vi "log_notifier.vi"(11 "NotifierReferences":T1) -> ()   [LabVIEW 2013]
doc: "Reads a log file and sends read data to the notifier once per second"
uses:
  Data/TypeDefs/Notifiers.ctl
  Data/TypeDefs/UTM Location.ctl
  Data/TypeDefs/Sail Set Suggestions.ctl
  Data/TypeDefs/Rudder Set Suggestions.ctl
  Data/TypeDefs/OverrideInformation.ctl
  Data/TypeDefs/OverrideMode.ctl
  Data/TypeDefs/MotorSetup.ctl
  Data/TypeDefs/DynamixelSetupInfo.ctl
  Data/TypeDefs/AirmarStatus.ctl
  Data/TypeDefs/HardwareOnline.ctl
  Data/TypeDefs/DynamixelCycleTracker.ctl
  Data/TypeDefs/RC Input Values.ctl
  Logic/Classes/Waypoint/Waypoint.lvclass
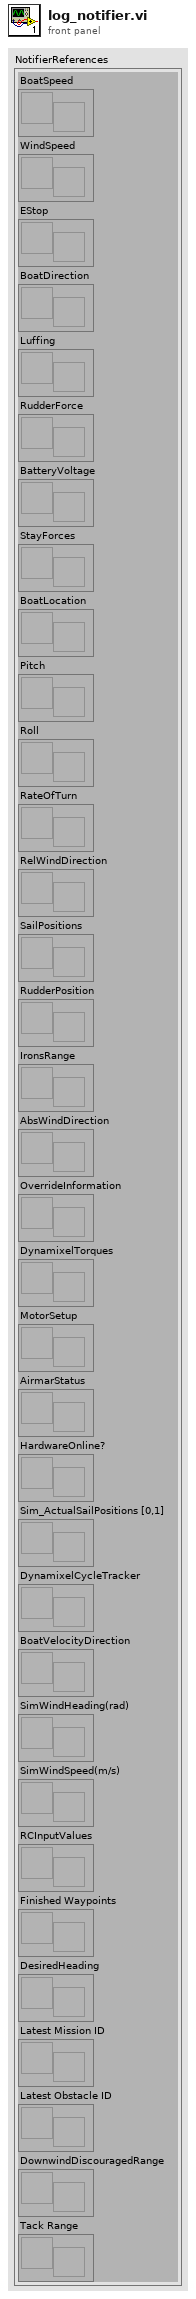
[diagram p1: front panel]
types:
  T1 = typedef "Notifiers.ctl" = cluster{"BoatSpeed":refnum<notifier>, "WindSpeed":refnum<notifier>, "EStop":refnum<notifier>, "BoatDirection":refnum<notifier>, "Luffing":refnum<notifier>, "RudderForce":refnum<notifier>, "BatteryVoltage":refnum<notifier>, "StayForces":refnum<notifier>, "BoatLocation":refnum<notifier>, "Pitch":refnum<notifier>, "Roll":refnum<notifier>, "RateOfTurn":refnum<notifier>, "RelWindDirection":refnum<notifier>, "SailPositions":refnum<notifier>, "RudderPosition":refnum<notifier>, "IronsRange":refnum<notifier>, "AbsWindDirection":refnum<notifier>, "OverrideInformation":refnum<notifier>, "DynamixelTorques":refnum<notifier>, "MotorSetup":refnum<notifier>, "AirmarStatus":refnum<notifier>, "HardwareOnline?":refnum<notifier>, "Sim_ActualSailPositions [0,1]":refnum<notifier>, "DynamixelCycleTracker":refnum<notifier>, "BoatVelocityDirection":refnum<notifier>, "SimWindHeading(rad)":refnum<notifier>, "SimWindSpeed(m/s)":refnum<notifier>, "RCInputValues":refnum<notifier>, "Finished Waypoints":refnum<notifier>, "DesiredHeading":refnum<notifier>, "Latest Mission ID":refnum<notifier>, "Latest Obstacle ID":refnum<notifier>, "DownwindDiscouragedRange":refnum<notifier>, "Tack Range":refnum<notifier>}
  T2 = typedef "BasicLogReading.ctl" = cluster{"BoatSpeed":dbl, "WindSpeed":dbl, "BoatDirection":dbl, "RelWindDirection":dbl, "AbsWindDirection":dbl, "SailPositions":T3, "RudderPosition":T4, "BoatLocation":T5}
  T3 = typedef "Sail Set Suggestions.ctl" = cluster{"MainSailSuggestion":dbl, "JibSailSuggestion":dbl}
  T4 = typedef "Rudder Set Suggestions.ctl" = dbl
  T5 = typedef "UTM Location.ctl" = cluster{"UTM Zone":dbl, "Hemisphere":enum16{"North", "South"}, "East":dbl, "North":dbl}
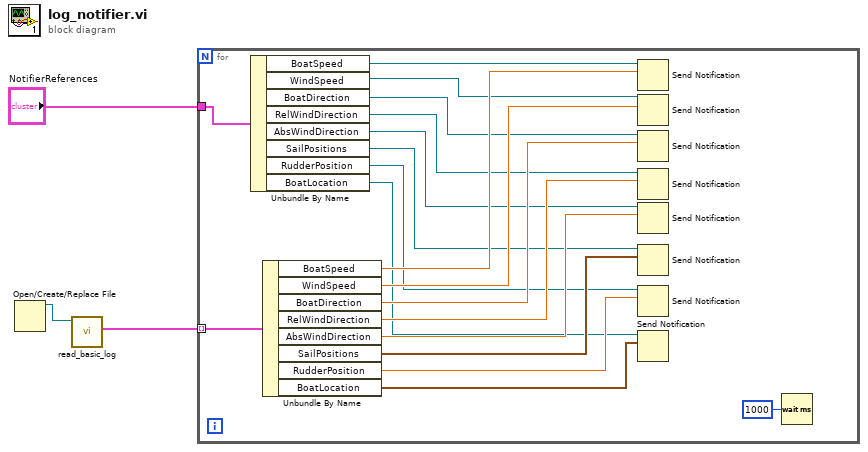
[diagram p0: block diagram]
diagram:
  n1 = Open/Create/Replace File() -> (refnum out=w3:refnum<file>)  [unwired: 6 in, 2 out]
  n2 = call "read_basic_log.vi"("refnum out"=w3) -> ("Array of gathered data in a cluster"=w2:T2[])  [unwired: 9 in, 1 out]
  n3 = for {
    tunnel: w2 -> [w22] mode=indexing
    tunnel: "NotifierReferences" -> [w21]
    n4 = Unbundle By Name(w21) -> ("BoatSpeed"=w20:refnum<notifier>, "WindSpeed"=w18:refnum<notifier>, "BoatDirection"=w16:refnum<notifier>, "RelWindDirection"=w14:refnum<notifier>, "AbsWindDirection"=w12:refnum<notifier>, "SailPositions"=w10:refnum<notifier>, "RudderPosition"=w8:refnum<notifier>, "BoatLocation"=w6:refnum<notifier>)
    n5 = Unbundle By Name(w22) -> ("BoatSpeed"=w19:dbl, "WindSpeed"=w17:dbl, "BoatDirection"=w15:dbl, "RelWindDirection"=w13:dbl, "AbsWindDirection"=w11:dbl, "SailPositions"=w9:T3, "RudderPosition"=w7:T4, "BoatLocation"=w5:T5)
    n6 = Send Notification(notification=w19, notifier=w20) -> ()  [unwired: 1 in, 2 out]
    n7 = Send Notification(notification=w17, notifier=w18) -> ()  [unwired: 1 in, 2 out]
    n8 = Send Notification(notification=w15, notifier=w16) -> ()  [unwired: 1 in, 2 out]
    n9 = Send Notification(notification=w13, notifier=w14) -> ()  [unwired: 1 in, 2 out]
    n10 = Send Notification(notification=w11, notifier=w12) -> ()  [unwired: 1 in, 2 out]
    n11 = Send Notification(notification=w9, notifier=w10) -> ()  [unwired: 1 in, 2 out]
    n12 = Send Notification(notification=w7, notifier=w8) -> ()  [unwired: 1 in, 2 out]
    n13 = Send Notification(notification=w5, notifier=w6) -> ()  [unwired: 1 in, 2 out]
    n14 = Wait (ms)(milliseconds to wait=u32 1000) -> ()  [unwired: 1 out]
  }
